vi "OAT CIC Decimation (Single Stage).vi"(6 "initial state":dbl[](array[numeric]), 7 "reset? (True)":bool=TRUE, 8 "error in (no error)":errorcluster, 10 "CIC filter settings":T1, 11 "X":dbl[](array[numeric]) format="%.2f") -> (0 "error out":errorcluster, 3 "Y":dbl[](array[numeric]) format="%.2f", 4 "final state":dbl[](array[numeric]))   [LabVIEW 2017, in "SoundVib_Resampling.lvlib"]
uses:
  <vilib>/addons/Sound and Vibration/Order Analysis/Resample Order Tracking/SoundVib_Resampling.lvlib
  <resource>/sndvib.dll
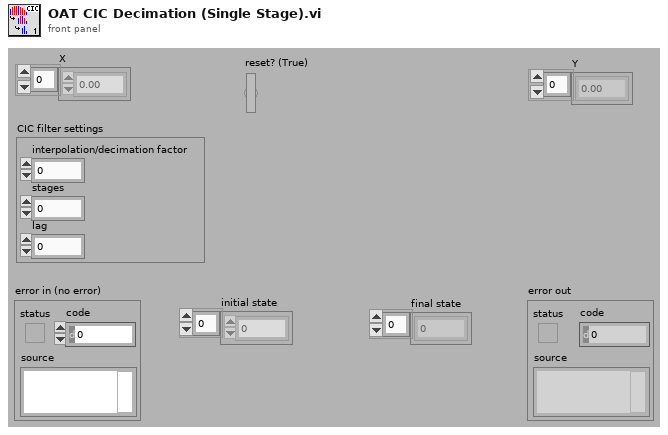
[diagram p1: front panel]
types:
  T1 = cluster{"interpolation/decimation factor":i32, "stages":i32, "lag":i32}
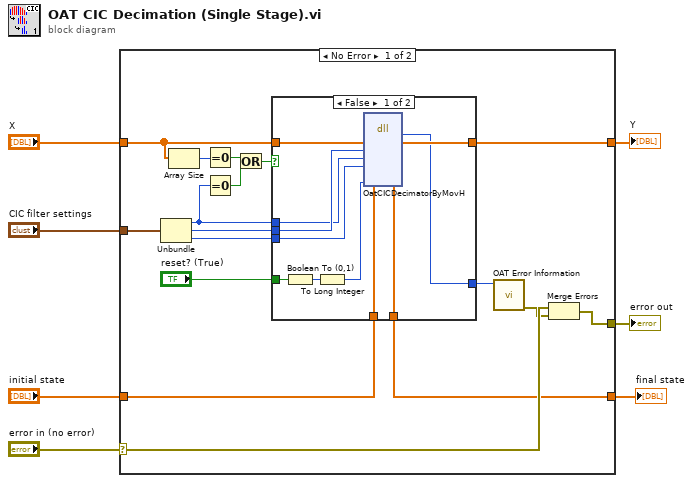
[diagram p0: block diagram]
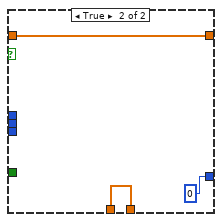
[diagram p2: hidden frame]
diagram:
  n1 = case shown="No Error" "error in (no error)" {
    selector: "error in (no error)" -> [w21 w40]
    tunnel: "X" -> [w24 w41]
    tunnel: [w23 w41] -> w6
    tunnel: [w22 w40] -> w5
    tunnel: "CIC filter settings" -> [w11 _]
    tunnel: "initial state" -> [w10 w39]
    tunnel: [w9 w39] -> w1
    frame No Error {
      n2 = Unbundle(w11) -> ("interpolation/decimation factor"=w18:i32, "stages"=w20:i32, "lag"=w19:i32)
      n3 = Array Size(array=w24) -> (size(s)=w15:i32)
      n4 = Equal To 0?(x=w15) -> (x = 0?=w14:bool)
      n5 = Equal To 0?(x=w18) -> (x = 0?=w13:bool)
      n6 = Or(x=w14, y=w13) -> (x .or. y?=w12:bool)
      n7 = case shown="False" w12 {
        tunnel: w24 -> [w35 w38]
        tunnel: [w29 w38] -> w23
        tunnel: w20 -> [w34 _]
        tunnel: w19 -> [w33 _]
        tunnel: w18 -> [w32 _]
        tunnel: w10 -> [w31 w36]
        tunnel: [w30 w36] -> w9
        tunnel: [w28 0] -> w17
        tunnel: "reset? (True)" -> [w27 _]
        frame False {
          n8 = Boolean To (0,1)(Boolean=w27) -> (0, 1=w26:i16)
          n9 = To Long Integer(number=w26) -> (32bit integer=w25:i32)
          n10 = dll-call lib="C:/Program Files (x86)/National Instruments/LabVIEW 2017/resource/sndvib.*" fn="OatCICDecimatorByMovH"("xH"=w35, "stage"=w34, "dec_factor"=w32, "lag"=w33, "initH"=w31, "reset"=w25) -> ("return type"=w28:i32, "xH"=w29:dbl[], "initH"=w30:dbl[])  [unwired: 7 in, 2 out]
        }
        frame True {
        }
      }
      n11 = call <vilib>:"OAT Error Information.vi"("error code"=w17) -> ("error out"=w8:errorcluster)  [unwired: 6 in]
      n12 = Merge Errors(w21, w8) -> (w22:errorcluster)
    }
    frame Error {
    }
  }
  "Y" <- w6
  "error out" <- w5
  "final state" <- w1
